vi "HSDIO Test.vi"() -> ()   [LabVIEW 2010]
uses:
  <vilib>/eio/EIONode/EIONode.xnode
  <vilib>/rvi/eio/nirviEIOImplementation/nirviEIOImplementation.xnode
  <vilib>/rvi/eio/common/nirviEmuClasses.ctl
  <vilib>/eio/EIOMethodNode/EIOMethodNode.xnode
  <vilib>/rvi/eio/nirviEIOMethodImplementation/nirviEIOMethodImplementation.xnode
  <vilib>/rvi/eio/common/nirviEmuTemplateMethod_noerrors.vi
panel:
  out "Ready":bool
  out "Rx":bool
  in  "Count(mSec)":u32
  in  "Wait?":bool
  in  "stop 2":bool
  out "Lidar Cable Check":bool
  out "Heartbeat":bool
  in  "stop":bool
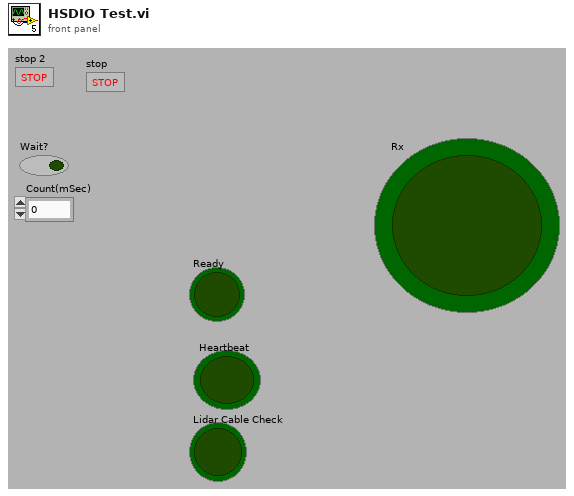
[diagram p1: front panel]
types:
  T1 = typedef "nirviEmuClasses.ctl" = enum16{"IO Read", "IO Write", "Method", "Property Read", "Property Write"}
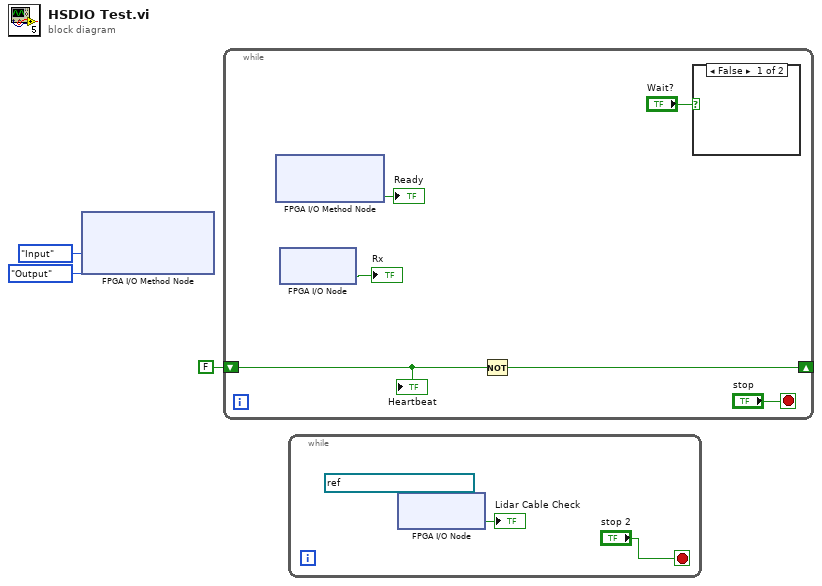
[diagram p0: block diagram]
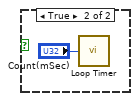
[diagram p2: hidden frame]
diagram:
  n1 = xnode "FPGA I/O Method Node"("DIO 7:4"=enum8{"No Change", "Input", "Output"}."Input", "DIO 3:0"=enum8{"No Change", "Input", "Output"}."Output") -> ()  [unwired: 1 in, 1 out]
  n2 = while {
    shift-right: [w7] -> _
    shift-left: FALSE -> [w8]
    stop <- "stop" stop-if-true
    n3 = xnode "FPGA I/O Method Node"() -> ("Ready"=→"Ready":bool)  [unwired: 1 in, 1 out]
    n4 = xnode "FPGA I/O Node"() -> ("Rx"=→"Rx":bool)  [unwired: 1 in, 1 out]
    n5 = Not(x=w8) -> (.not. x?=w7:bool)
    n6 = case shown="False" "Wait?" {
      frame False {
      }
      frame True {
        n7 = call "Loop Timer"("Count(mSec)"="Count(mSec)") -> ()  [unwired: 1 out]
      }
    }
    "Heartbeat" <- w8
  }
  n8 = while {
    stop <- "stop 2" stop-if-true
    n9 = xnode "FPGA I/O Node"("FPGA I/O In"=refnum<k21> "Lidar Data Cable Check") -> ("I/O Item"=→"Lidar Cable Check":bool)  [unwired: 1 out]
  }
